vi "DFT 512 (SubVI).vi"(10 "DFT  size in":i32=-1, 11 "Datos":dbl[](array[numeric])) -> (1 "DFT  size out":i32, 2 "x":i32, 3 "Array":dbl[](array[numeric]))   [LabVIEW 2020]
uses:
  <vilib>/Analysis/2dsp.llb/Real FFT.vi
  <vilib>/Analysis/NI_AALPro.lvlib
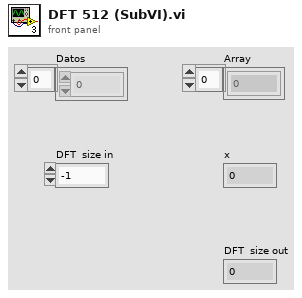
[diagram p1: front panel]
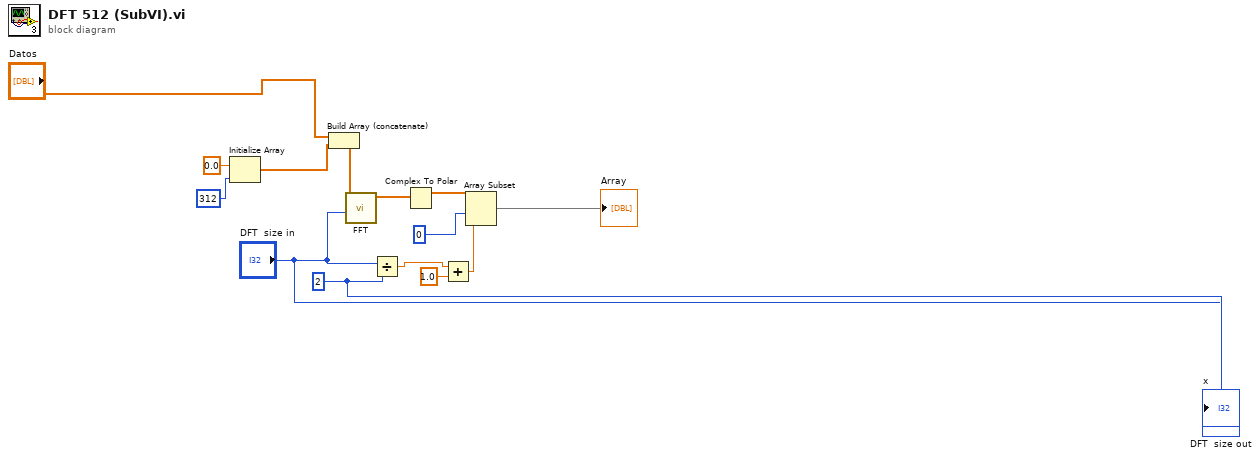
[diagram p0: block diagram]
diagram:
  w12 = 2 ("x")
  n1 = Initialize Array(0.0 ("element"), 312 ("dimension size")) -> (w10:dbl[])
  n2 = Build Array (concatenate)("Datos", w10) -> (w7:dbl[])
  n3 = call-poly <vilib>:"FFT.vi"("FFT size"="DFT  size in", "X"=w7) -> ("FFT {X}"=w1:cdb[])  [unwired: 8 in, 1 out]
  n4 = Divide(x="DFT  size in", y=w12) -> (x/y=w3:dbl)
  n5 = Complex To Polar(r * e^(i*theta)=w1) -> (r=w2:dbl[])  [unwired: 1 out]
  n6 = Add(x=w3, y=1.0) -> (x+y=w4:dbl)
  n7 = Array Subset(array=w2, index=0, length=w4) -> (→"Array":dbl[])
  "x" <- w12
  "DFT  size out" <- "DFT  size in"
